vi "Stop Core.vi"(10 "final error code":i32, 11 "EMS Generic in":refnum<class "EMS Generic.lvclass">) -> (3 "EMS Generic out":refnum<class "EMS Generic.lvclass">)   [LabVIEW 2018, in "EMS Generic Actor.lvlib" / "EMS Generic.lvclass"]
doc: "(<B>Filename</B>: Actor Framework.lvlib:Actor.lvclass:Stop Core.vi)\n\nDefines what the actor does before it stops. Use the <B>final error code</B> input to determine whether the actor shut down in response to an error.\n\nBy default, this method does nothing. A descendant class may override it to define behavior, such as shutting down any processes the actor initiated in its override of the Actor Core method."
uses:
  EMS Generic.lvclass
  EMS Generic.lvclass/EMS Generic.ctl
  <vilib>/ActorFramework/Actor/Actor.lvclass
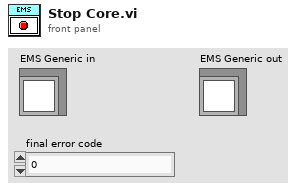
[diagram p1: front panel]
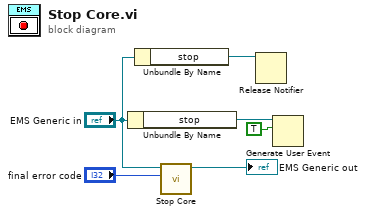
[diagram p0: block diagram]
diagram:
  n1 = Unbundle By Name("EMS Generic in") -> ("stop"=w3:refnum<user-event>)
  n2 = Unbundle By Name("EMS Generic in") -> ("stop"=w1:refnum<notifier>)
  n3 = call-parent "Stop Core.vi"("final error code"="final error code", "Actor in"="EMS Generic in") -> ("Actor out"=→"EMS Generic out":refnum<class "EMS Generic.lvclass">)  [unwired: 9 in]
  n4 = Release Notifier(notifier=w1) -> ()  [unwired: 2 in, 3 out]
  n5 = Generate User Event(user event=w3, event data cluster=TRUE ("event data")) -> ()  [unwired: 2 in, 2 out]
